vi "Method.vi"(4 "Numeric":refnum<class "Abs_Numeric.lvclass">) -> (1 "Result":refnum<class "Abs_Double Float.lvclass">)   [LabVIEW 2021, in "Reciprocal_Numeric.lvclass"]
uses:
  Reciprocal_Numeric.lvclass
  Abs_Types/Double Float/Abs_Double Float.lvclass
  Abs_Types/Numeric/Abs_Numeric.lvclass
  C:/Program Files (x86)/National Instruments/LabVIEW 2021/vi.lib/TSA/Abstract Data Classes/Abs_Types/Double Float/Abs_Double Float.lvclass
  Reciprocal_Numeric.lvclass/Reciprocal_Numeric.ctl
  Properties/Write Numeric.vi
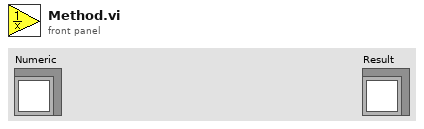
[diagram p1: front panel]
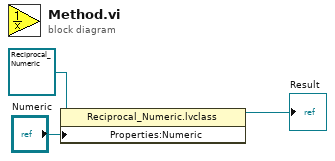
[diagram p0: block diagram]
diagram:
  n1 = property class="Reciprocal_Numeric.lvclass"(reference=refnum<class "Reciprocal_Numeric.lvclass"> refnum ("Decrement_DBL.lvclass"), "Properties:Numeric"="Numeric") -> (reference out=→"Result":refnum<class "Reciprocal_Numeric.lvclass">)  [unwired: 1 in, 1 out]
